vi "getSampleInfo.vi"(8 "error in (no error)":errorcluster, 10 "times":dbl[](array[numeric]), 11 "SoundDeviceData in":refnum<class "SoundDeviceData.lvclass">) -> (0 "error out":errorcluster, 1 "sampleRate":dbl, 2 "sampleNumber":i32, 3 "SoundDeviceData out":refnum<class "SoundDeviceData.lvclass">)   [LabVIEW 2011, in "DataMappers.lvlib" / "SoundDeviceData.lvclass"]
uses:
  SoundDeviceData.lvclass
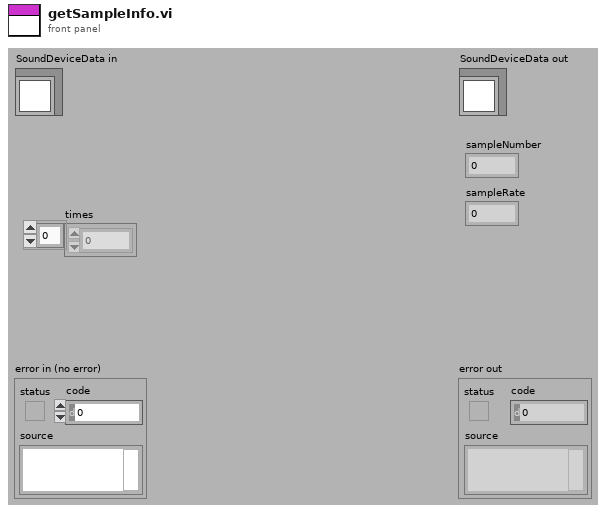
[diagram p1: front panel]
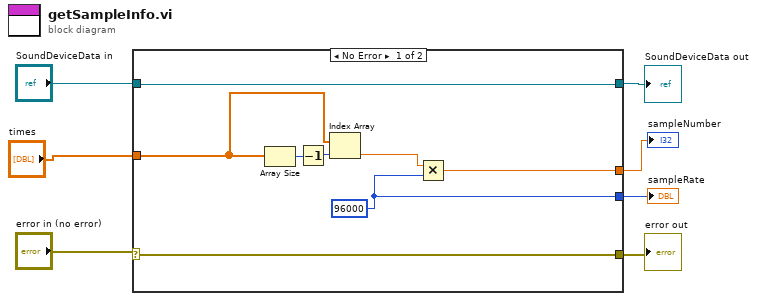
[diagram p0: block diagram]
diagram:
  n1 = case shown="No Error" "error in (no error)" {
    selector: "error in (no error)" -> [w9 w16]
    tunnel: [w10 w17] -> w6
    tunnel: "SoundDeviceData in" -> [w10 w17]
    tunnel: [w9 w16] -> w4
    tunnel: [w12 _] -> w3
    tunnel: [w11 _] -> w2
    tunnel: "times" -> [w8 _]
    frame No Error {
      w11 = 96000
      n2 = Array Size(array=w8) -> (size(s)=w15:i32)
      n3 = Decrement(x=w15) -> (x-1=w14:i32)
      n4 = Index Array(array=w8, index=w14) -> (element=w13:dbl)
      n5 = Multiply(x=w13, y=w11) -> (x*y=w12:dbl)
    }
    frame Error {
    }
  }
  "error out" <- w4
  "SoundDeviceData out" <- w6
  "sampleNumber" <- w3
  "sampleRate" <- w2
